vi "XML File.vi"(9 "Action":T1) -> (1 "Output":string)   [LabVIEW 2020, in "NIVS_Consolidated_CDW_MetaDataObj.lvclass"]
doc: "Constants, which are necessary for the custom device <B>XML file</B>."
uses:
  NIVS_Consolidated_CDW_MetaDataObj.lvclass
  XML File.ctl
  Common.ctl
  Common.vi
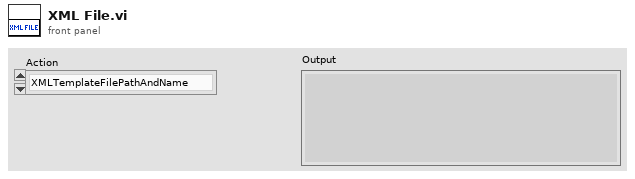
[diagram p1: front panel]
types:
  T1 = typedef "NIVS_Consolidated_CDW_MetaDataObj.lvclass/XML File.ctl" = enum16{"XMLTemplateFilePathAndName", "XMLTimingAndSyncFileName", "XMLCustomDeviceFileName", "XMLTemplateFilePathAndName (Inline-Async)", "XMLPPLTemplateFilePathAndName (Inline-Async)", "XMLPPLTemplateFilePathAndName (Inline)"}
  T2 = typedef "NIVS_Consolidated_CDW_MetaDataObj.lvclass/Common.ctl" = enum16{"ProjectName", "TemplatesFolderName", "PPLTemplatesFolderName", "ProjectTemplatePathAndName", "ProjectPPLTemplatePathAndName", "TimingAndSyncFolderName", "CustomDeviceFolderName", "PathToTemplates", "PathToPPLTemplates", "PathToExplorerPPLTemplates", "PathToEnginePPLTemplates", "PathToConfigurationFile", "ProjectConfigurationName"}
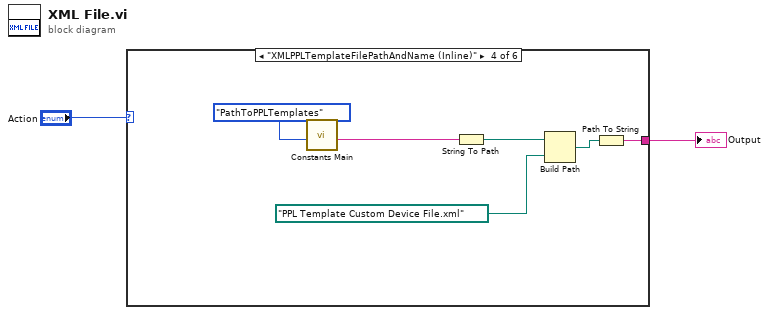
[diagram p0: block diagram]
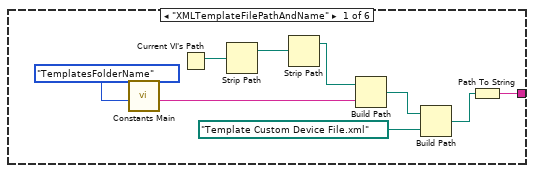
[diagram p2: hidden frame]
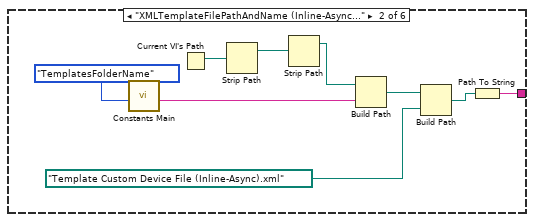
[diagram p3: hidden frame]
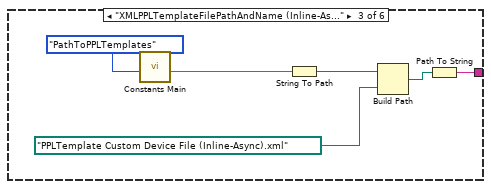
[diagram p4: hidden frame]
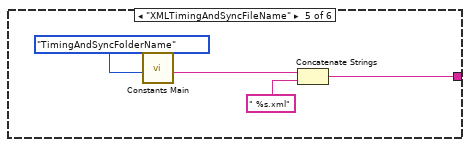
[diagram p5: hidden frame]
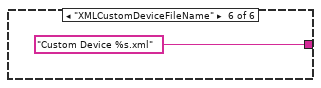
[diagram p6: hidden frame]
diagram:
  n1 = case shown="\"XMLPPLTemplateFilePathAndName (Inline)\"" "Action" {
    tunnel: [w9 w18 w25 w31 w33 "Custom Device %s.xml" ("format string")] -> w2
    frame "XMLTemplateFilePathAndName" {
      n2 = call-poly "Constants Main.vi"("Action"=Common."TemplatesFolderName") -> ("Output"=w10:string)  [unwired: 10 in]
      n3 = Current VI's Path() -> (path=w5:path)
      n4 = Strip Path(path=w5) -> (stripped path=w4:path)  [unwired: 1 out]
      n5 = Strip Path(path=w4) -> (stripped path=w3:path)  [unwired: 1 out]
      n6 = Build Path(base path=w3, name or relative path=w10) -> (appended path=w8:path)
      n7 = Build Path(base path=w8, name or relative path=path "Template Custom Device File.xml" ("format string")) -> (appended path=w6:path)
      n8 = Path To String(path=w6) -> (string=w9:string)
    }
    frame "XMLTemplateFilePathAndName (Inline-Async)" {
      n9 = call-poly "Constants Main.vi"("Action"=Common."TemplatesFolderName") -> ("Output"=w19:string)  [unwired: 10 in]
      n10 = Current VI's Path() -> (path=w14:path)
      n11 = Strip Path(path=w14) -> (stripped path=w13:path)  [unwired: 1 out]
      n12 = Strip Path(path=w13) -> (stripped path=w12:path)  [unwired: 1 out]
      n13 = Build Path(base path=w12, name or relative path=w19) -> (appended path=w17:path)
      n14 = Build Path(base path=w17, name or relative path=path "Template Custom Device File (Inline-Async).xml" ("format string")) -> (appended path=w15:path)
      n15 = Path To String(path=w15) -> (string=w18:string)
    }
    frame "XMLPPLTemplateFilePathAndName (Inline-Async)" {
      n16 = call-poly "Constants Main.vi"("Action"=Common."PathToPPLTemplates") -> ("Output"=w22:string)  [unwired: 10 in]
      n17 = String To Path(string=w22) -> (path=w21:path)
      n18 = Build Path(base path=w21, name or relative path=path "PPLTemplate Custom Device File (Inline-Async).xml" ("format string")) -> (appended path=w23:path)
      n19 = Path To String(path=w23) -> (string=w25:string)
    }
    frame "XMLPPLTemplateFilePathAndName (Inline)" {
      n20 = call-poly "Constants Main.vi"("Action"=Common."PathToPPLTemplates") -> ("Output"=w28:string)  [unwired: 10 in]
      n21 = String To Path(string=w28) -> (path=w27:path)
      n22 = Build Path(base path=w27, name or relative path=path "PPL Template Custom Device File.xml" ("format string")) -> (appended path=w29:path)
      n23 = Path To String(path=w29) -> (string=w31:string)
    }
    frame "XMLTimingAndSyncFileName" {
      n24 = call-poly "Constants Main.vi"("Action"=Common."TimingAndSyncFolderName") -> ("Output"=w35:string)  [unwired: 10 in]
      n25 = Concatenate Strings(w35, " %s.xml" ("format string")) -> (w33:string)
    }
    frame "XMLCustomDeviceFileName" {
    }
  }
  "Output" <- w2
